vi "OEE_MAIN_set_config_info.vi"(10 "Array":string[](array[string]), 11 "SQL_raw_data_in":T1) -> (3 "SQL_raw_data_out":T1)   [LabVIEW 2019]
uses:
  FGV/SQL_raw_data/OEE_SQL_raw_data.ctl
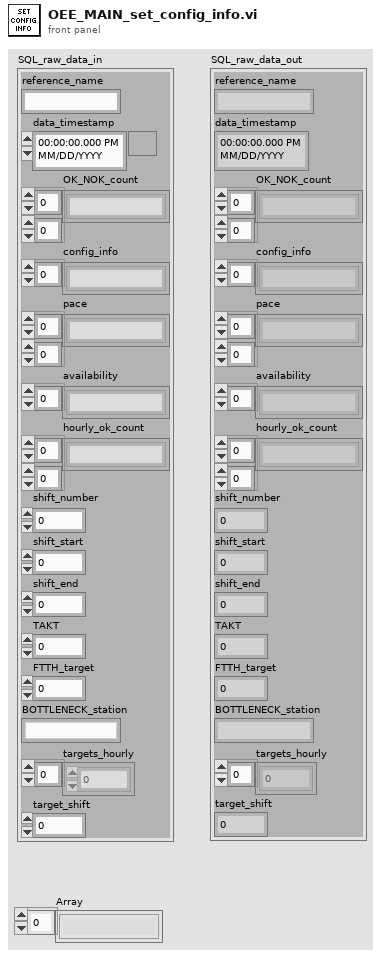
[diagram p1: front panel]
types:
  T1 = typedef "OEE_SQL_raw_data.ctl" = cluster{"reference_name":string, "data_timestamp":timestamp, "OK_NOK_count":string[][], "config_info":string[], "pace":string[][], "availability":string[], "hourly_ok_count":string[][], "shift_number":i8, "shift_start":i8, "shift_end":i8, "TAKT":u16, "FTTH_target":u16, "BOTTLENECK_station":string, "targets_hourly":u16[], "target_shift":u16}
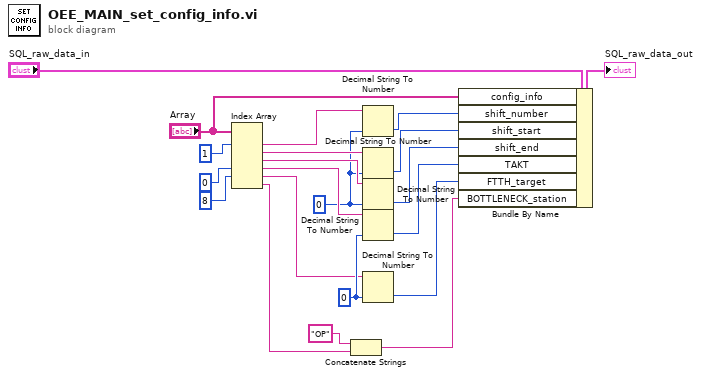
[diagram p0: block diagram]
diagram:
  w21 = u16 0 ("default (0 I32)")
  w2 = i8 0 ("default (0 I32)")
  n1 = Index Array(array="Array", index #1=1 ("index"), index #4=0 ("index"), index #5=8 ("index")) -> (element #1=w3:string, element #2=w13:string, element #3=w14:string, element #4=w18:string, element #5=w8:string, element #6=w7:string)  [unwired: 3 in]
  n2 = Concatenate Strings("OP" ("string"), w7) -> (w5:string)
  n3 = Decimal String To Number(string=w3, default (0L)=w2) -> (number=w1:i8)  [unwired: 1 in, 1 out]
  n4 = Decimal String To Number(string=w13, default (0L)=w2) -> (number=w16:i8)  [unwired: 1 in, 1 out]
  n5 = Decimal String To Number(string=w14, default (0L)=w2) -> (number=w15:i8)  [unwired: 1 in, 1 out]
  n6 = Decimal String To Number(string=w18, default (0L)=w21) -> (number=w19:u16)  [unwired: 1 in, 1 out]
  n7 = Decimal String To Number(string=w8, default (0L)=w21) -> (number=w20:u16)  [unwired: 1 in, 1 out]
  n8 = Bundle By Name(cluster="SQL_raw_data_in", "config_info"="Array", "shift_number"=w1, "shift_start"=w16, "shift_end"=w15, "TAKT"=w19, "FTTH_target"=w20, "BOTTLENECK_station"=w5) -> (→"SQL_raw_data_out":T1)
